vi "offsetXY.vi"(6 "Thres":dbl, 9 "Previous":dbl[][](array[numeric]), 10 "Current":dbl[][](array[numeric])) -> (1 "OffsetY":dbl, 2 "OffsetX":dbl)   [LabVIEW 2011]
panel:
  out "x > y?":bool
  out "Current 2":dbl[][](array[numeric])
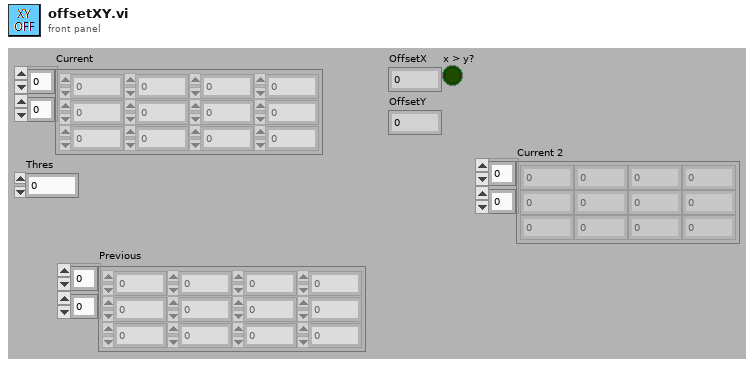
[diagram p1: front panel]
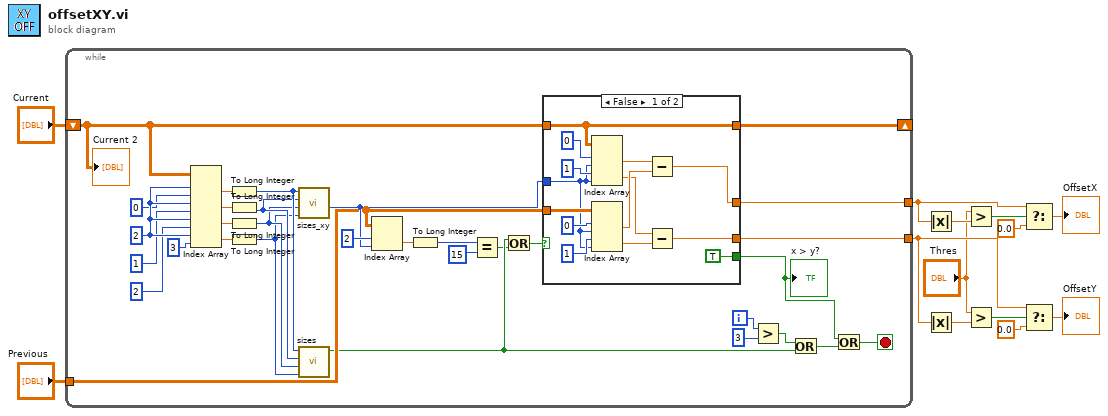
[diagram p0: block diagram]
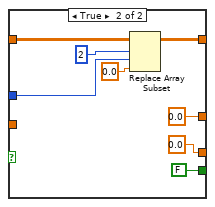
[diagram p2: hidden frame]
diagram:
  n1 = while {
    tunnel: "Previous" -> [w30]
    shift-right: [w29] -> _
    shift-left: "Current" -> [w32]
    tunnel: [w26] -> w2
    tunnel: [w25] -> w8
    i -> [w28]
    stop <- w23 stop-if-true
    w45 = 2 ("index (row)")
    n2 = Index Array(array=w32, index (row) #1=w45, index (col) #1=0 ("disabled index (col)"), index (row) #2=w45, index (col) #2=1 ("disabled index (col)"), index (row) #3=w45, index (col) #3=2 ("disabled index (col)"), index (row) #4=w45, index (col) #4=3 ("disabled index (col)")) -> (element #1=w40:dbl, element #2=w39:dbl, element #3=w38:dbl, element #4=w37:dbl)
    n3 = To Long Integer(number=w40) -> (32bit integer=w22:i32)
    n4 = To Long Integer(number=w39) -> (32bit integer=w21:i32)
    n5 = To Long Integer(number=w38) -> (32bit integer=w20:i32)
    n6 = To Long Integer(number=w37) -> (32bit integer=w19:i32)
    n7 = call "sizes_xy.vi"("Size 4"=w19, "Size 3"=w20, "Size 2"=w21, "Size 1"=w22) -> ("led 1"=w31:i32)  [unwired: 7 in]
    n8 = call "sizes.vi"("Size 4"=w19, "Size 3"=w20, "Size 2"=w21, "Size 1"=w22) -> ("Problem"=w16:bool)  [unwired: 5 in, 2 out]
    n9 = Index Array(array=w30, index (row)=2 ("disabled index (row)"), index (col)=w31) -> (element=w34:dbl)
    n10 = To Long Integer(number=w34) -> (32bit integer=w33:i32)
    n11 = Equal?(x=w33, y=15) -> (x = y?=w15:bool)
    n12 = Or(x=w16, y=w15) -> (x .or. y?=w14:bool)
    n13 = case shown="False" w14 {
      tunnel: w32 -> [w49 w67]
      tunnel: w31 -> [w53 w66]
      tunnel: [w49 w63] -> w29
      tunnel: w30 -> [w55 _]
      tunnel: [w48 0.0 ("new element/subarray")] -> w26
      tunnel: [w47 0.0 ("new element/subarray")] -> w25
      tunnel: [TRUE ("x > y?") FALSE ("x > y?")] -> w24
      frame False {
        n14 = Index Array(array=w49, index (row) #1=0 ("index (row)"), index (col) #1=w53, index (row) #2=1 ("index (row)"), index (col) #2=w53) -> (element #1=w54:dbl, element #2=w51:dbl)
        n15 = Index Array(array=w55, index (row) #1=0 ("index (row)"), index (col) #1=w53, index (row) #2=1 ("index (row)"), index (col) #2=w53) -> (element #1=w52:dbl, element #2=w50:dbl)
        n16 = Subtract(x=w54, y=w52) -> (x-y=w48:dbl)
        n17 = Subtract(x=w51, y=w50) -> (x-y=w47:dbl)
      }
      frame True {
        n18 = Replace Array Subset(array=w67, new element=0.0 ("new element/subarray"), index (row)=2 ("disabled index (row)"), index (col)=w66) -> (w63:dbl[][])
      }
    }
    "x > y?" <- w24
    n19 = Greater?(x=w28, y=3) -> (0:w18:bool)
    n20 = Or(x=w18, y=w16) -> (x .or. y?=w17:bool)
    n21 = Or(x=w24, y=w17) -> (x .or. y?=w23:bool)
    "Current 2" <- w32
  }
  n22 = Absolute Value(x=w2) -> (abs(x)=w5:dbl)
  n23 = Absolute Value(x=w8) -> (abs(x)=w10:dbl)
  n24 = Greater?(x="Thres", y=w5) -> (0:w6:bool)
  n25 = Greater?(x="Thres", y=w10) -> (0:w11:bool)
  n26 = Select(t=w2, s=w6, f=0.0) -> (s? t:f=→"OffsetX":dbl)
  n27 = Select(t=w8, s=w11, f=0.0) -> (s? t:f=→"OffsetY":dbl)
